vi "DatabaseHand_Group_Get(string).vi"(8 "error in (no error)":errorcluster, 10 "group":string, 11 "Database RefNum in":T1) -> (0 "error out":errorcluster, 1 "group string":string, 2 "group array":string[][](array[string]), 3 "Database RefNum out":T1)   [LabVIEW 2016]
doc: "This VI finds the RefNum of an existing object with the input Name or creates a new object if the Name is not found or Name is unwired or an empty string.\nCopyright 2001 VI Engineering, Inc."
uses:
  private/vis/DatabaseHand_RefNum.ctl
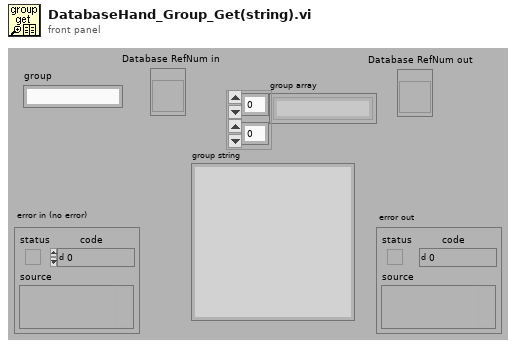
[diagram p1: front panel]
types:
  T1 = typedef "DatabaseHand_RefNum.ctl" = refnum<vi>
  T2 = typedef "DatabaseHan_DatabaseElement.ctl" = cluster{"name":string, "value":string, "type":string, "unit":string, "permissions":string, "enqueued":bool, "group":string}
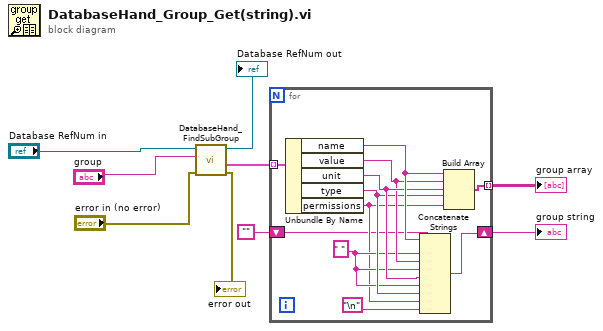
[diagram p0: block diagram]
diagram:
  n1 = call "DatabaseHand_FindSubGroup.vi"("error in (no error)"="error in (no error)", "group"="group", "Database RefNum in"="Database RefNum in") -> ("error out"=→"error out":errorcluster, "group found"=w6:T2[], "Database RefNum out"=→"Database RefNum out":T1)  [unwired: 6 out]
  n2 = for {
    tunnel: w6 -> [w20] mode=indexing
    tunnel: [w19] -> w5 mode=indexing
    shift-right: [w11] -> w3
    shift-left: "" -> [w10]
    w14 = " "
    n3 = Unbundle By Name(w20) -> ("name"=w18:string, "value"=w16:string, "unit"=w17:string, "type"=w15:string, "permissions"=w13:string)
    n4 = Concatenate Strings(w10, w18, w14, w16, w14, w17, w14, w15, w13, "\n") -> (w11:string)
    n5 = Build Array(w18, w16, w17, w15, w13) -> (w19:string[])
  }
  "group array" <- w5
  "group string" <- w3
